vi "VGLOBAL.vi"() -> ()   [LabVIEW 2021]
panel:
  in  "GLOBAL04STOP":bool
  in  "GLOBAL.03STOP":bool
  out "GLOBAL02LED":bool
  in  "GLOBAL01DBL":dbl
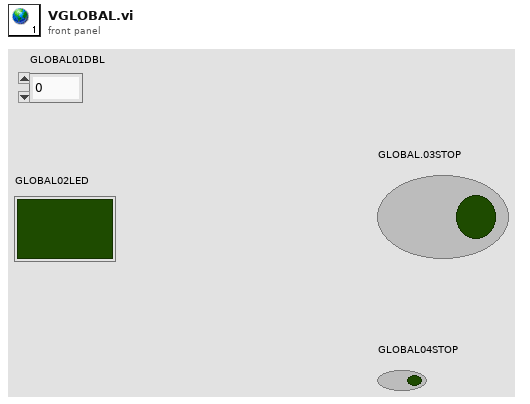
[diagram p1: front panel]
diagram:
